vi "ActionVIOnLoad.vi"(8 "error in (no error)":errorcluster, 11 "Device Item Ref in":T1 format="%.0x") -> (0 "error out":errorcluster, 3 "Device Item Ref out":T1 format="%.0x")   [LabVIEW 2015, in "OPC UA Client System Explorer.lvlib"]
uses:
  OPC UA Client System Explorer.lvlib
  <vilib>/NI Veristand/Custom Device API/Custom Device Item Ref.ctl
  NationalInstruments.VeriStand.SystemDefinitionAPI
  Shared/Constants.vi
  <vilib>/NI VeriStand/Custom Device API/Custom Device API.lvlib
  Shared/OPC UA Client Shared.lvlib
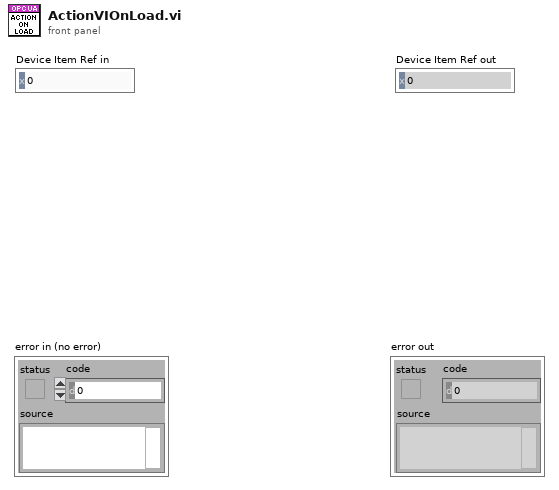
[diagram p1: front panel]
types:
  T1 = typedef "Custom Device API.lvlib/Custom Device Item Ref.ctl" = u64
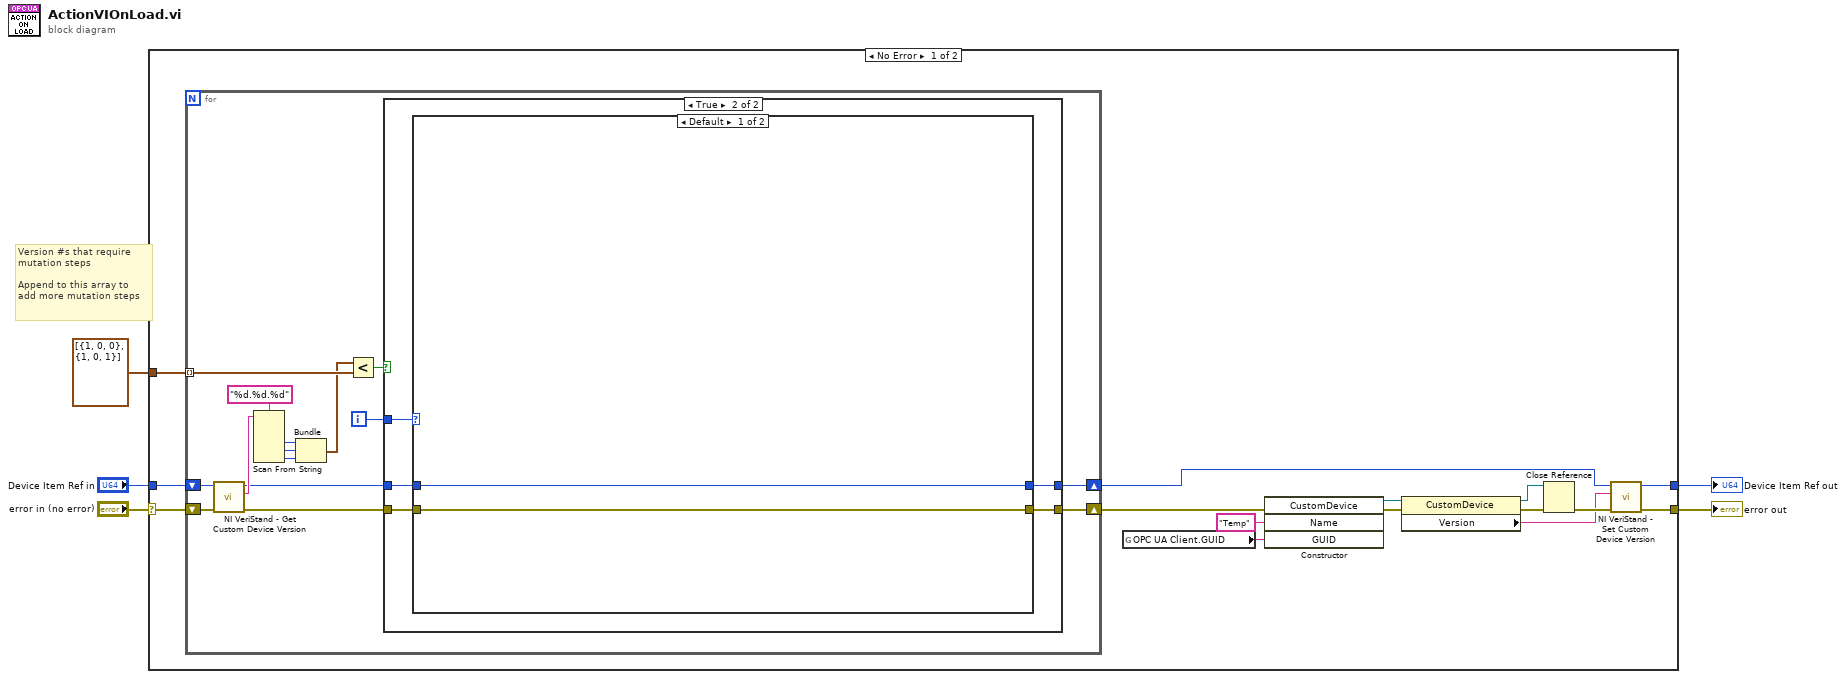
[diagram p0: block diagram]
diagram:
  # "Version #s that require\nmutation steps\n\nAppend to this array to\nadd more mutation steps"
  n1 = case shown="No Error" "error in (no error)" {
    selector: "error in (no error)" -> [w19 w48]
    tunnel: [w11 w48] -> w2
    tunnel: "Device Item Ref in" -> [w18 w47]
    tunnel: [w10 w47] -> w1
    tunnel: cluster{i32, i32, i32}[] [{1, 0, 0}, {1, 0, 1}] -> [w20 _]
    frame No Error {
      n2 = for {
        tunnel: w20 -> [w23] mode=indexing
        shift-right: [w28] -> w9
        shift-left: w19 -> [w33]
        shift-right: [w26] -> w8
        shift-left: w18 -> [w32]
        i -> [w25]
        n3 = call <vilib>:"NI VeriStand - Get Custom Device Version.vi"("error in (no error)"=w33, "Device Ref in"=w32) -> ("error out"=w29:errorcluster, "Value"=w31:string, "Device Ref out"=w27:T1)  [unwired: 7 in]
        n4 = Scan From String(format string="%d.%d.%d", input string=w31) -> (output 1=w34:i32, output 2=w35:i32, output 3=w22:i32)  [unwired: 5 in, 3 out]
        n5 = Bundle(w34, w35, w22) -> (w21:cluster{i32, i32, i32})  [unwired: 1 in]
        n6 = Less?(x=w21, y=w23) -> (x < y?=w30:bool)
        n7 = case shown="True" w30 {
          tunnel: w29 -> [w37 w42]
          tunnel: [w37 w41] -> w28
          tunnel: w27 -> [w36 w38]
          tunnel: [w36 w39] -> w26
          tunnel: w25 -> [_ w40]
          frame False {
          }
          frame True {
            n8 = case shown="Default" w40 {
              tunnel: w42 -> [w44 w46]
              tunnel: [w44 w46] -> w41
              tunnel: [w43 w45] -> w39
              tunnel: w38 -> [w43 w45]
              frame Default {
              }
              frame 0 {
              }
            }
          }
        }
      }
      n9 = global read "Constants.vi" "OPC UA Client.GUID"() -> (w6:string)
      n10 = constructor class="CustomDevice"(error in=w9, "Name"="Temp", "GUID"=w6) -> (reference out=w17:refnum<k24>, error out=w16:errorcluster)  [unwired: 2 in, 3 out]
      n11 = property class="CustomDevice"(reference=w17, error in=w16) -> (reference out=w14:refnum<k24>, error out=w15:errorcluster, "Version"=w12:string)
      n12 = Close Reference(reference=w14, error in (no error)=w15) -> (error out=w13:errorcluster)
      n13 = call <vilib>:"NI VeriStand - Set Custom Device Version.vi"("error in (no error)"=w13, "Value"=w12, "Device Ref in"=w8) -> ("error out"=w11:errorcluster, "Device Ref out"=w10:T1)  [unwired: 7 in]
    }
    frame Error {
    }
  }
  "error out" <- w2
  "Device Item Ref out" <- w1
